vi "Read-Write.vi"() -> ()   [LabVIEW 2016]
uses:
  <vilib>/Analysis/2dsp.llb/Real FFT.vi
  <vilib>/Analysis/NI_AALPro.lvlib
panel:
  in  "Start":dbl
  out "FFT":dbl[](graph)
  in  "N":i32=-1
  in  "Path 2":path
  out "Output":waveform(dbl)(graph)
  out "sampling rate":dbl
  out "Input":waveform(dbl)(graph)
  in  "Path":path
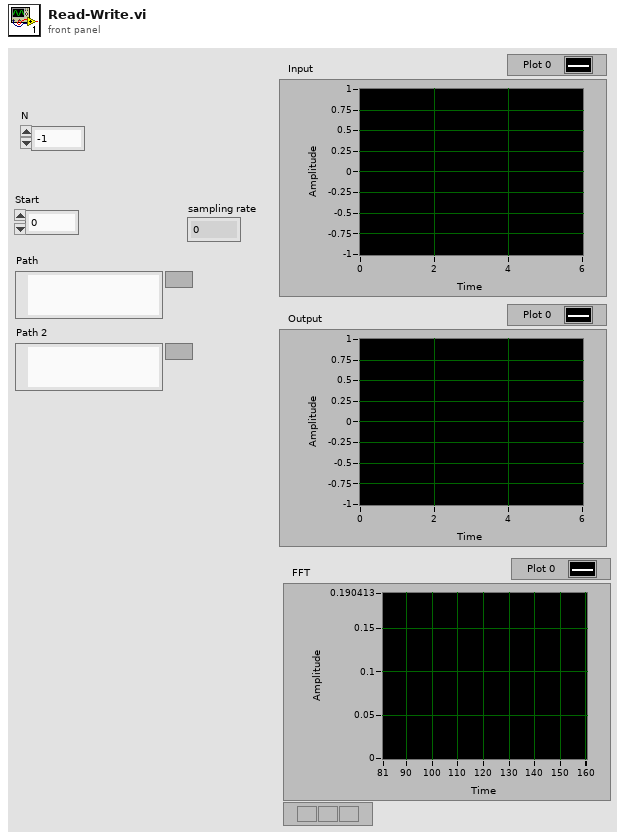
[diagram p1: front panel]
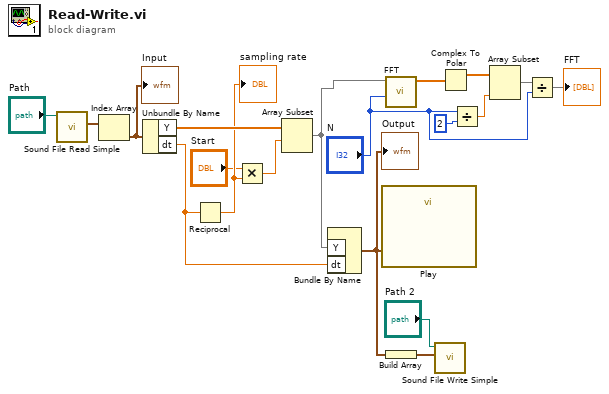
[diagram p0: block diagram]
diagram:
  n1 = call <vilib>:"Sound File Read Simple.vi"("path"="Path") -> ("data"=w19:waveform(dbl)[])  [unwired: 7 in, 3 out]
  n2 = Index Array(array=w19) -> (element=w18:waveform(dbl))  [unwired: 1 in]
  "Input" <- w18
  n3 = Unbundle By Name(w18) -> ("Y"=w12:dbl[], "dt"=w13:dbl)
  n4 = Reciprocal(x=w13) -> (1/x=w11:dbl)
  "sampling rate" <- w11
  n5 = Multiply(x="Start", y=w11) -> (x*y=w10:dbl)
  n6 = Array Subset(array=w12, index=w10) -> (w1:dbl[])  [unwired: 1 in]
  n7 = Bundle By Name("Y"=w1, "dt"=w13) -> (w16:waveform(dbl))  [unwired: 1 in]
  "Output" <- w16
  n8 = call "Play"("Data"=w16) -> ()  [unwired: 18 in, 1 out]
  n9 = call-poly <vilib>:"FFT.vi"("FFT size"="N", "X"=w1) -> ("FFT {X}"=w9:cdb[])  [unwired: 8 in, 1 out]
  n10 = Build Array(w16) -> (w15:waveform(dbl)[])
  n11 = call <vilib>:"Sound File Write Simple.vi"("data"=w15, "path"="Path 2") -> ()  [unwired: 8 in, 2 out]
  n12 = Complex To Polar(r * e^(i*theta)=w9) -> (r=w8:dbl[])  [unwired: 1 out]
  n13 = Divide(x="N", y=2) -> (x/y=w6:dbl)
  n14 = Array Subset(array=w8, length=w6) -> (w5:dbl[])  [unwired: 1 in]
  n15 = Divide(x=w5, y="N") -> (x/y=→"FFT":dbl[])
